vi "direct_ads_sur_T_pw.vi"(8 "Error (Input)":errorcluster, 9 "Loading in kg/kg (Input)":dbl, 10 "Pressure in Pa (Input)":dbl, 11 "WorkingPair (Input)":T1={"no_iso"=1, "no_p_sat"=1, "path_db"="D:\\Driesel\\SorpLibLocal\\LabVIEW_wrapper\\data\\json\\sorpproplib_minimalExample.json", "wp_as"="silicagel", "wp_st"="123", "wp_iso"="DubininArctan1", "wp_rf"="water", "rf_rhol"="SaturatedLiquidDensity_EoS1", "no_rhol"=1, "rf_psat"="VaporPressure_EoS1"}) -> (0 "Error (Output)":errorcluster caption="Error(Output)", 3 "Temperature in K (Output)":dbl)   [LabVIEW 2017]
doc: "direct_ads_sur_T_pw:\n * --------------------\n *\n * Calculates equilibrium temperature in K depending on equilibrium pressure p\n * in Pa, equilibrium loading w in kg/kg, and specified working pair.\n *\n * Parameters:\n * -----------\n * double p_Pa:\n * Equilibrium pressure in Pa.\n * double w_kgkg:\n * Equilibrium loading in kg/kg.\n *\n * const char *path_db:\n * Path to database.\n * const char *wp_as:\n * Name of sorbent.\n * const char *wp_st:\n * Name of sub-type of sorbent.\n * const char *wp_rf:\n * Name of refrigerant.\n * const char *wp_iso:\n * Name of isotherm.\n * int no_iso:\n * ID of isotherm (i.e. when more than one isotherm is available)\n * const char *rf_psat:\n * Name of calculation approach for vapor pressure.\n * int no_p_sat:\n * ID of vapor pressure equation (i.e. when more than one equation is\n * available)\n * const char *rf_rhol:\n * Name of calculation approach for liquid density.\n * int no_rhol:\n * ID of liquid density equation (i.e. when more than one equation is\n * available)\n * Name of calculation approach for liquid density.\n *\n * Returns:\n * --------\n * double:\n * Equilibrium temperature in K.\n *\n * Remarks:\n * --------\n * This function is only valid for isotherm models based on the surface\n * approach.\n *\n * History:\n * --------\n * 07/07/2021, by Jannik Driesel (supervised by Mirko Engelpracht):\n * First implementation."
uses:
  data/win32bit/libsorpPropLib.dll
panel:
  # "Path to database"
  # "Name of sorbent"
  # "Name of sub-type of sorbent"
  # "Name of refrigerant"
  # "Name of isotherm"
  # "ID of isotherm"
  # "Name of calculation approach for vapor pressure"
  # "ID of vapor pressure equation"
  # "Name of calculation approach for liquid density"
  # "ID of liquid density equation"
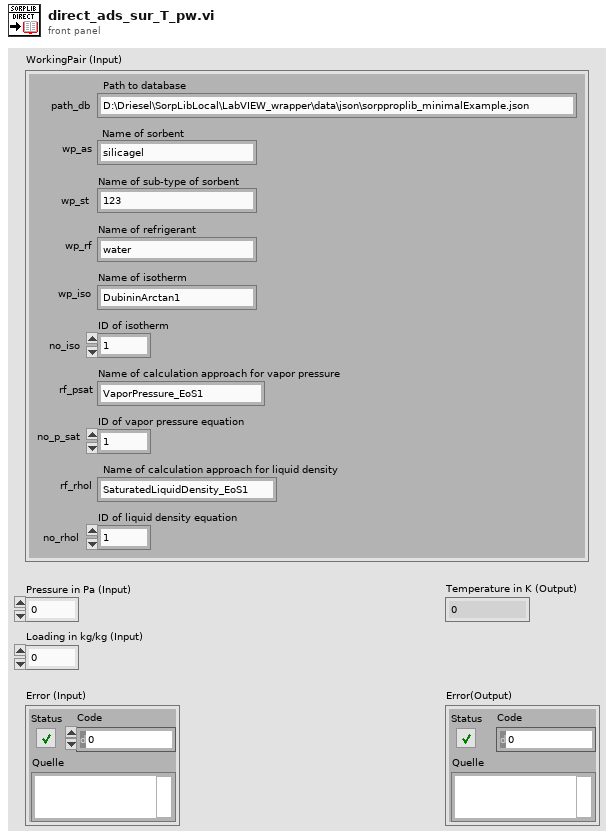
[diagram p1: front panel]
types:
  T1 = cluster{"no_iso":i32, "no_p_sat":i32, "path_db":string, "wp_as":string, "wp_st":string, "wp_iso":string, "wp_rf":string, "rf_rhol":string, "no_rhol":i32, "rf_psat":string}
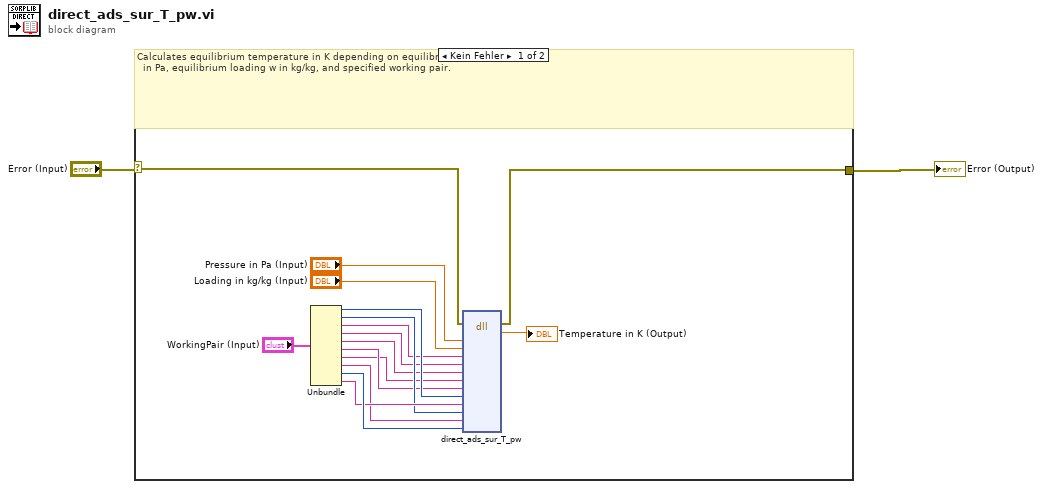
[diagram p0: block diagram]
diagram:
  n1 = case shown="Kein Fehler" "Error (Input)" {
    selector: "Error (Input)" -> [w6 w19]
    tunnel: [w5 w19] -> w1
    frame No Error {
      # "Calculates equilibrium temperature in K depending on equilibrium pressure p\n  in Pa, equilibrium loading w in kg/kg, and specified working pair."
      n2 = Unbundle("WorkingPair (Input)") -> ("no_iso"=w14:i32, "no_p_sat"=w15:i32, "path_db"=w8:string, "wp_as"=w9:string, "wp_st"=w10:string, "wp_iso"=w12:string, "wp_rf"=w11:string, "rf_rhol"=w13:string, "no_rhol"=w17:i32, "rf_psat"=w16:string)
      n3 = dll-call lib="D:/Driesel/SorpLibLocal/LabVIEW_wrapper/data/win32bit/libsorpPropLib.dll" fn="direct_ads_sur_T_pw"(error in=w6, "p_Pa"="Pressure in Pa (Input)", "w_kgkg"="Loading in kg/kg (Input)", "path_db"=w8, "wp_as"=w9, "wp_st"=w10, "wp_rf"=w11, "wp_iso"=w12, "no_iso"=w14, "rf_psat"=w16, "no_p_sat"=w15, "rf_rhol"=w13, "no_rhol"=w17) -> (error out=w5:errorcluster, "T_K"=→"Temperature in K (Output)":dbl)  [unwired: 14 in, 1 out]
    }
    frame Error {
      # "Error - No calculations"
    }
  }
  "Error (Output)" <- w1
